vi "Configure and Query the Auto Range.vi"(5 "Enable to Query":bool=TRUE, 7 "Enable to Sets":bool=TRUE, 8 "error in":errorcluster, 9 "Sets the Auto Range":u16(ring) items=["Auto Range Off", "Auto Range On"], 10 "Sets to Display":u16(ring) items=["1st Display", "2nd Display"], 11 "VISA resource name":refnum<visa-resource-name>) -> (0 "error out":errorcluster, 2 "Return the Auto Range status":string, 3 "VISA resource name out":refnum<visa-resource-name>)   [LabVIEW 2011, in "DMM4.lvlib"]
uses:
  <instrlib>/DMM4/DMM4.lvlib
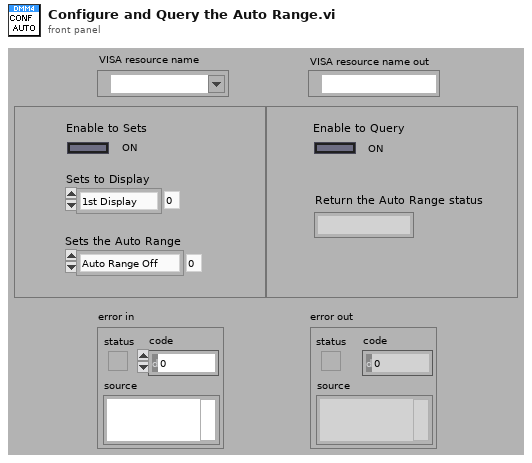
[diagram p1: front panel]
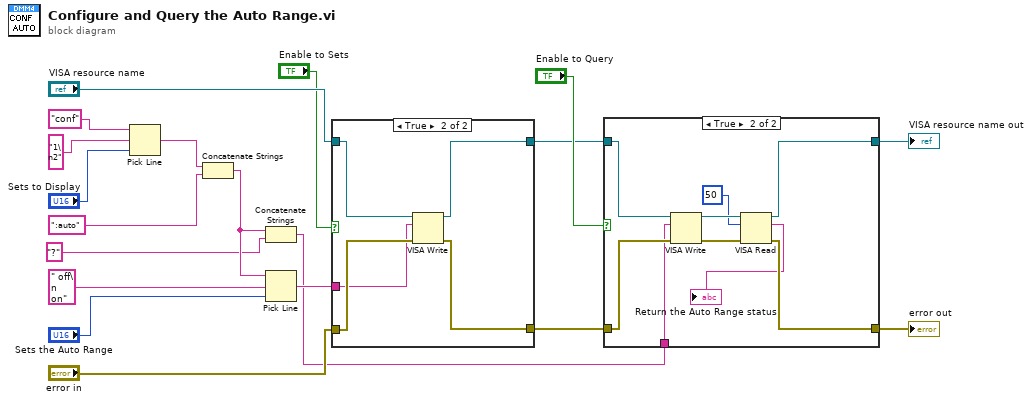
[diagram p0: block diagram]
diagram:
  n1 = Pick Line(string ("")="conf", multi-line string="1\n2", line index="Sets to Display") -> (output string=w16:string)
  n2 = Concatenate Strings(w16, ":auto") -> (w12:string)
  n3 = Concatenate Strings(w12, "?") -> (w1:string)
  n4 = Pick Line(string ("")=w12, multi-line string=" off\n on", line index="Sets the Auto Range") -> (output string=w8:string)
  n5 = case shown="True" "Enable to Sets" {
    tunnel: "VISA resource name" -> [w21 w26]
    tunnel: "error in" -> [w20 w25]
    tunnel: w8 -> [_ w24]
    tunnel: [w21 w23] -> w5
    tunnel: [w20 w22] -> w4
    frame False {
    }
    frame True {
      n6 = VISA Write(VISA resource name=w26, write buffer=w24, error in (no error)=w25) -> (VISA resource name out=w23:refnum<visa-resource-name>, error out=w22:errorcluster)  [unwired: 1 out]
    }
  }
  n7 = case shown="True" "Enable to Query" {
    tunnel: w5 -> [w27 w34]
    tunnel: w4 -> [w28 w33]
    tunnel: [w28 w31] -> w2
    tunnel: [w27 w32] -> w3
    tunnel: w1 -> [_ w29]
    frame False {
    }
    frame True {
      n8 = VISA Write(VISA resource name=w34, write buffer=w29, error in (no error)=w33) -> (VISA resource name out=w37:refnum<visa-resource-name>, error out=w36:errorcluster)  [unwired: 1 out]
      n9 = VISA Read(VISA resource name=w37, byte count=u32 50, error in (no error)=w36) -> (VISA resource name out=w32:refnum<visa-resource-name>, read buffer=→"Return the Auto Range status":string, error out=w31:errorcluster)  [unwired: 1 out]
    }
  }
  "VISA resource name out" <- w3
  "error out" <- w2
